vi "test_serialize_deserialize.vi"   [LabVIEW 2020, in "ADAS_Data_Type_Template.lvlib"]
doc: "Version 0.1"
uses:
  ADAS_Data_Type_Template.lvlib
  <vilib>/addons/_JKI Toolkits/Caraya/classes/Test/Test.lvclass
  <vilib>/addons/_JKI Toolkits/Caraya/classes/Assert/Assert.lvclass
  Process Data.ctl
  CustomDataTypes/ADAS Generic/Serialize Data.vi
  CustomDataTypes/ADAS Generic/NI_ADAS_Generic.lvlib
  CustomDataTypes/ADAS Generic/Deserialize Data.vi
types:
  T1 = typedef "ADAS_Data_Type_Template.lvlib/Process Data.ctl" = cluster{}
  T2 = typedef "NI_ADAS_Generic.lvlib/Process Data.ctl" = cluster{"Timestamp":timestamp, "Bus Channel":u16, "Byte Array":u8[]}
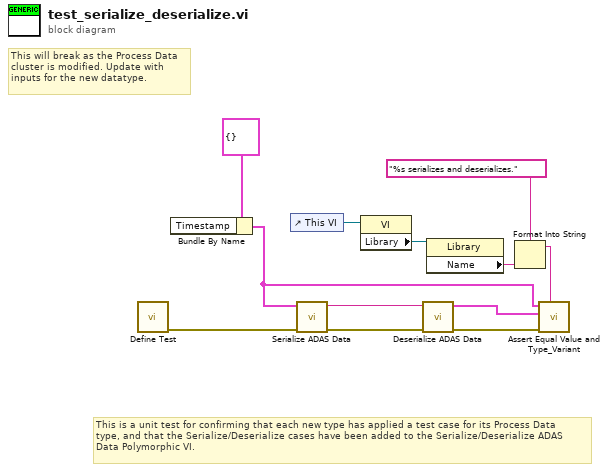
[diagram p0: block diagram]
diagram:
  # "This will break as the Process Data\ncluster is modified. Update with\ninputs for the new datatype."
  # "This is a unit test for confirming that each new type has applied a test case for its Process Data\ntype, and that the Serialize/Deserialize cases have been added to the Serialize/Deserialize ADAS\nData Polymorphic VI."
  n1 = call <vilib>:"Define Test.vi"() -> ("error out"=w7:errorcluster)  [unwired: 11 in]
  n2 = Bundle By Name "Bundle By Name"(cluster=T1 {} ("Process Data in")) -> (w1:T1)  [unwired: 1 in]
  n3 = control-ref of="This VI"() -> (w12:refnum<vi>)
  n4 = call-poly "Serialize ADAS Data.vi"("error in (no error)"=w7, "Process Data"=w1) -> ("error out"=w6:errorcluster, "Flat Data out"=w5:string)  [unwired: 8 in]
  n5 = property class="VI"(reference=w12) -> ("Library"=w11:refnum<vi>)  [unwired: 1 in, 2 out]
  n6 = call-poly "Deserialize ADAS Data.vi"("error in (no error)"=w6, "Flat Data in"=w5) -> ("error out"=w3:errorcluster, "Process Data out"=w4:T2)  [unwired: 8 in]
  n7 = property class="Library"(reference=w11) -> ("Name"=w9:string)  [unwired: 1 in, 2 out]
  n8 = Format Into String(format string="%s serializes and deserializes.", w9) -> (resulting string=w8:string)  [unwired: 2 in, 1 out]
  n9 = call <vilib>:"Assert Equal Value and Type_Variant.vi"("Label"=w8, "error in (no error)"=w3, "Y"=w4, "X"=w1) -> ()  [unwired: 7 in, 1 out]
